vi "Stop Core.vi"(8 "error in (no error)":errorcluster, 11 "Halfwave Fit Display in":refnum<class "Halfwave Fit Display.lvclass">) -> (0 "error out":errorcluster, 3 "Halfwave Fit Display out":refnum<class "Halfwave Fit Display.lvclass">)   [LabVIEW 2016, in "Halfwave Fit Display.lvclass"]
uses:
  Halfwave Fit Display.lvclass
  Halfwave Fit Display.lvclass/Halfwave Fit Display.ctl
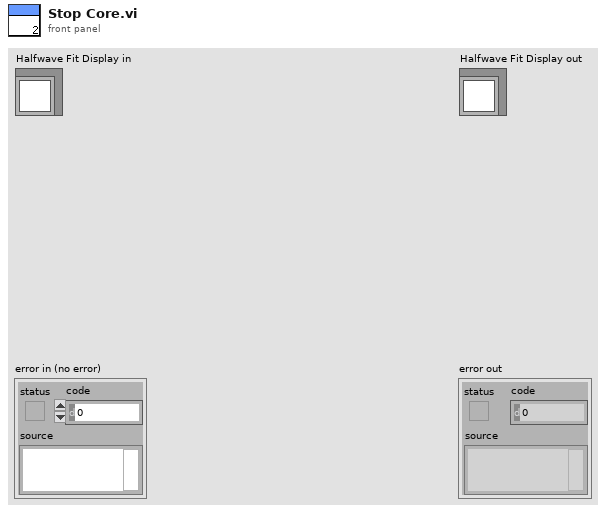
[diagram p1: front panel]
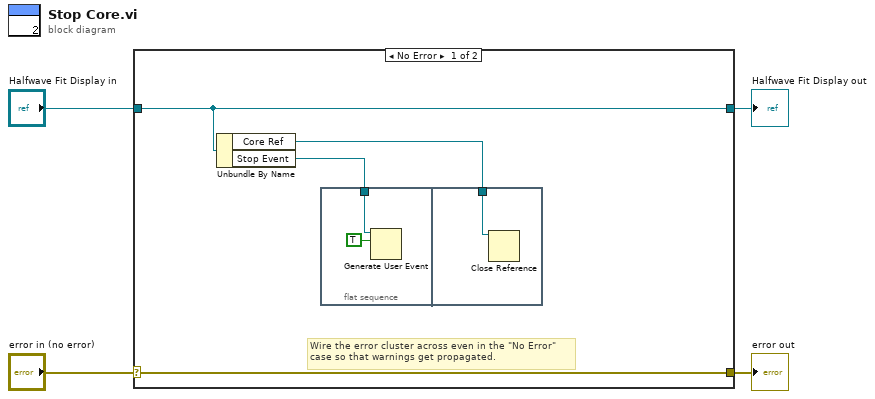
[diagram p0: block diagram]
diagram:
  n1 = case shown="No Error" "error in (no error)" {
    selector: "error in (no error)" -> [w8 w13]
    tunnel: [w8 w13] -> w3
    tunnel: [w7 w12] -> w1
    tunnel: "Halfwave Fit Display in" -> [w7 w12]
    frame No Error {
      # "Wire the error cluster across even in the \"No Error\"\ncase so that warnings get propagated."
      n2 = Unbundle By Name(w7) -> ("Core Ref"=w5:refnum<vi>, "Stop Event"=w6:refnum<user-event>)
      n3 = flat-sequence {
        tunnel: w6 -> [w10]
        tunnel: w5 -> [w11]
        frame #0 {
          n4 = Generate User Event(user event=w10, event data cluster=TRUE ("event data")) -> ()  [unwired: 2 in, 2 out]
        }
        frame #1 {
          n5 = Close Reference(reference=w11) -> ()  [unwired: 1 in, 1 out]
        }
      }
    }
    frame Error {
    }
  }
  "error out" <- w3
  "Halfwave Fit Display out" <- w1
